vi "TPNT_CheckIfRegister.vi"(10 "value in":string) -> (2 "value out":string)   [LabVIEW 2016]
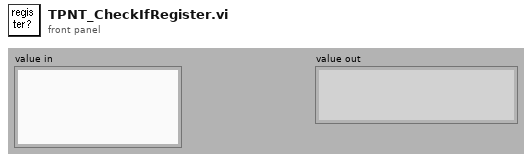
[diagram p1: front panel]
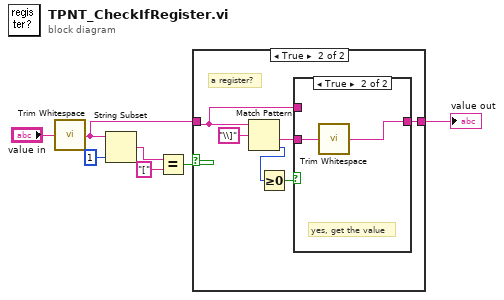
[diagram p0: block diagram]
diagram:
  n1 = call <vilib>:"Trim Whitespace.vi"("string"="value in") -> ("trimmed string"=w2:string)  [unwired: 1 in]
  n2 = String Subset(string=w2, length (rest)=1 ("length (rest)")) -> (substring=w5:string)  [unwired: 1 out]
  n3 = Equal?(x=w5, y="[") -> (x = y?=w3:bool)
  n4 = case shown="True" w3 {
    tunnel: w2 -> [w8 w11]
    tunnel: [w8 w10] -> w1
    frame False {
      # "not a register"
    }
    frame True {
      # "a register?"
      n5 = Match Pattern(string=w11, regular expression="\\]") -> (after substring=w9:string, offset past match=w13:i32)  [unwired: 3 out]
      n6 = Greater Or Equal To 0?(x=w13) -> (x >= 0?=w12:bool)
      n7 = case shown="True" w12 {
        tunnel: w11 -> [w15 _]
        tunnel: [w15 w16] -> w10
        tunnel: w9 -> [_ w17]
        frame False {
          # "nop, pass it"
        }
        frame True {
          # "yes, get the value"
          n8 = call <vilib>:"Trim Whitespace.vi"("string"=w17) -> ("trimmed string"=w16:string)  [unwired: 1 in]
        }
      }
    }
  }
  "value out" <- w1
